vi "VFH.vi"() -> ()   [LabVIEW 2016]
panel:
  out "VFH error":bool
  in  "Outer Thershold":dbl
  in  "Inner Threshold":dbl=0.420745
  in  "obstacle clearance distance":dbl=0.420745
  out "mask":bool[](array[boolean])
  out "histogram":dbl[](array[numeric])
  out "Distance":dbl[](array[numeric])
  out "Angle":dbl[](array[numeric])
  in  "Target Angle":dbl
  in  "출력 클러스터":T1
  in  "V_max":dbl
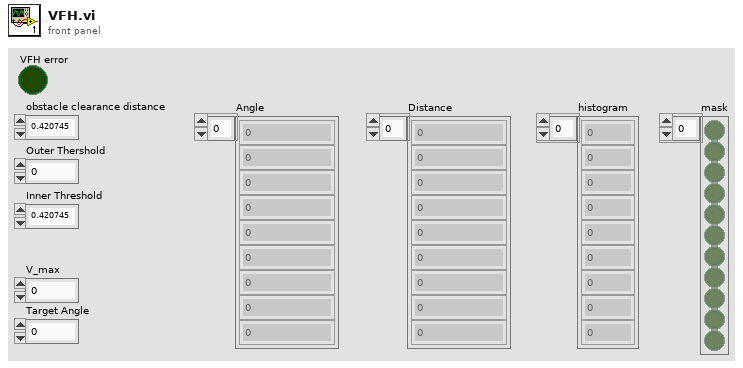
[diagram p1: front panel]
types:
  T1 = cluster{"Inner Thershold":dbl, "Outer Thershold":dbl}
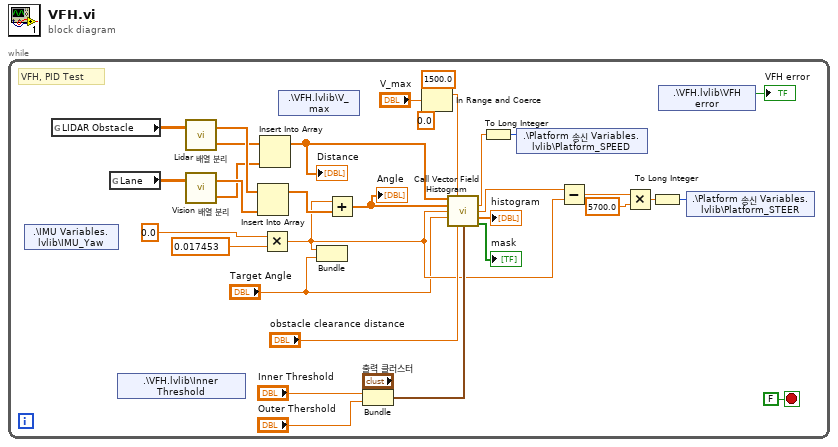
[diagram p0: block diagram]
diagram:
  n1 = while {
    stop <- FALSE stop-if-true
    # "VFH, PID Test"
    n2 = shared-variable ".\\IMU Variables.lvlib\\IMU_Yaw"() -> ()  [unwired: 1 in, 2 out]
    n3 = global read "[GV]_Lidar Obstacle.vi" "LIDAR Obstacle"() -> (w27:dbl[][])
    n4 = global read "[GV]_Vision Lane.vi" "Lane"() -> (w26:dbl[][])
    n5 = shared-variable ".\\VFH.lvlib\\Inner Threshold"() -> ()  [unwired: 1 in, 2 out]
    n6 = call "Lidar 배열 분리.vi"("행렬"=w27) -> ("Lidar Distance (m)"=w22:dbl[], "Lidar Angle (rad)"=w24:dbl[])  [unwired: 1 in]
    n7 = call "Vision 배열 분리.vi"("Vision Data"=w26) -> ("Vision Distance (m)"=w23:dbl[], "Vision Angle (rad)"=w25:dbl[])  [unwired: 1 in]
    n8 = Insert Into Array(array=w24, new element=w25) -> (w21:dbl[])  [unwired: 1 in]
    n9 = Insert Into Array(array=w22, new element=w23) -> (w15:dbl[])  [unwired: 1 in]
    "Distance" <- w15
    n10 = Multiply(x=0.0, y=0.017453 ("GPS_Longitude 2")) -> (x*y=w13:dbl)
    n11 = shared-variable ".\\VFH.lvlib\\V_max"() -> ()  [unwired: 1 in, 2 out]
    n12 = Bundle(w13, "Target Angle"="Target Angle") -> ()  [unwired: 1 in, 1 out]
    n13 = Add(x=w13, y=w21) -> (x+y=w14:dbl[])
    "Angle" <- w14
    n14 = Bundle(cluster="출력 클러스터", "Inner Thershold"="Inner Threshold", "Outer Thershold"="Outer Thershold") -> (w19:T1)
    n15 = In Range and Coerce(upper limit=1500.0 ("상위 리미트"), x="V_max", lower limit=0.0 ("하위 리미트")) -> (coerced(x)=w5:dbl)  [unwired: 1 out]
    n16 = call "Call Vector Field Histogram.vi"("LIDAR magn. (m)"=w15, "max speed (protocol)"=w5, "LIDAR angle (rad)"=w14, "current heading (rad)"=w13, "target heading (rad)"="Target Angle", "obstacle clearance (m)"="obstacle clearance distance", "thresholds"=w19) -> ("command speed (protocol)"=w10:dbl, "command heading (rad)"=w12:dbl, "histogram out"=→"histogram":dbl[], "mask out"=→"mask":bool[])  [unwired: 5 in]
    n17 = To Long Integer(number=w10) -> (32bit integer=w9:i32)
    n18 = shared-variable ".\\Platform 송신 Variables.lvlib\\Platform_SPEED"(w9) -> ()  [unwired: 1 in, 1 out]
    n19 = Subtract(x=w12, y=w13) -> (x-y=w28:dbl)
    n20 = Multiply(x=w28, y=5700.0) -> (x*y=w31:dbl)
    n21 = To Long Integer(number=w31) -> (32bit integer=w30:i32)
    n22 = shared-variable ".\\VFH.lvlib\\VFH error"() -> (→"VFH error":bool)  [unwired: 1 in, 1 out]
    n23 = shared-variable ".\\Platform 송신 Variables.lvlib\\Platform_STEER"(w30) -> ()  [unwired: 1 in, 1 out]
  }
